vi "encoder_test_3mode_2motor_2.vi"() -> ()   [LabVIEW 2014]
uses:
  <vilib>/rvi/FXPMathLib/FxpSinAndCos/subVIs/nifxpmath_SinAndCos_SimConfig.ctl
  <vilib>/rvi/Emulation/niFpgaGetClockAttributes.vi
  <vilib>/rvi/Emulation/niFpgaSctlEmulationGetInTimedLoop.vi
  <vilib>/rvi/Emulation/niFpgaEmulationReportErrorSimple.vi
  <vilib>/rvi/eio/common/nirviEmuTemplateMethod_errors.vi
  <vilib>/rvi/Emulation/niFpgaProcessEmulError.vi
  <vilib>/rvi/Emulation/niFpgaCriticalErrorInLSC.vi
  <vilib>/rvi/FXPMathLib/FxpSinAndCos/simVIs/DllFxpSinAndCosTemp_sub.vi
  <vilib>/rvi/interface/RandomDataEmulation/nirviRandomDataMultiElementFPGAFIFO.vi
  <instcachedir>/0/nirviRandomDataMultiElementFPGAFIFO_AD0CFC12EF974623A9C2E4184BC062B2.lvgen/nirviRandomDataMultiElementFPGAFIFO_AD0CFC12EF974623A9C2E4184BC062B2_023.vi
  <vilib>/rvi/interface/RandomDataEmulation/niFpgaRandomDataHandleErrors.vi
  <vilib>/eio/EIONode/EIONode.xnode
  <vilib>/rvi/FXPMathLib/FxpMul/XNode/nifxpmath_Multiplier.xnode
  <vilib>/rvi/FXPMathLib/FxpSinAndCos/XNode/nifxpmath_SinAndCos.xnode
  <vilib>/rvi/Analysis/measure/butterworth/XNode/niFpgaButterworthFilter.xnode
  <vilib>/rvi/FXPMathLib/FxpSub/XNode/nifxpmath_Sub.xnode
  <vilib>/rvi/FXPMathLib/FxpAdd/XNode/nifxpmath_Add.xnode
  <vilib>/rvi/DataTransferAndStorage/Container/XNode/niFpgaContainer.xnode
  <vilib>/rvi/interface/RandomDataEmulation/nirviRandomDataFpgaMultiElementTemplate.vi
  <vilib>/rvi/FXPMathLib/sim/FxpSim.dll
panel:
  in  "mt0_y":u32
  out "Dyr_sin_dd":fxp<+/-,64,25>
  out "Dyr_sin_d":fxp<+/-,64,16>
  out "Dyr_sin":fxp<+/-,30,11>
  in  "Sin offset_y":fxp<+/-,29,10>
  out "Sin omega_y":fxp<+/-,41,8>
  in  "Sin magnitude_y":fxp<+/-,11,8>
  in  "Sin frequency_y (Hz)":fxp<+/-,21,5>
  out "Dyr_ramp":fxp<+/-,32,7>
  out "Time now_y (s)":fxp<+,52,14>
  out "Dyr_slope":fxp<+/-,32,10>
  in  "Dyr_time":fxp<+/-,32,10>
  in  "Dyr_end":fxp<+/-,32,7>
  out "Dy_i":fxp<+/-,32,10>
  out "Dyr":fxp<+/-,36,11>
  in  "Direction_y":bool
  in  "Command type_y":i16(ring) items=["Step", "Ramp", "Sine"]
  out "Dy_error":fxp<+/-,37,10>
  out "Fmr_y":fxp<+/-,32,10>
  in  "Ki_y":fxp<+/-,20,6>
  in  "Dy_tolorence":fxp<+/-,18,1>
  in  "Kd_y":fxp<+/-,20,8>
  in  "Kp_y":fxp<+/-,20,8>
  in  "scaled coefficients_Dy_dd":i32[](array[numeric])=[780119100, 146811362]
  out "Dy_dd":fxp<+/-,36,10>
  out "va_y":fxp<+/-,38,8>
  out "vb_y":fxp<+/-,38,8>
  out "vd_y":fxp<+/-,20,5>
  out "vq_y":fxp<+/-,20,5> format="%.57g"
  in  "Stop motor_y":bool
  out "Dy_d (mm/s)":fxp<+/-,33,9>
  out "omega_y (rad/s)":fxp<+/-,33,9>
  in  "Velocity Estimation_y":i16(ring) items=["M_avg method", "M method", "T method"]
  out "Dy_d (T)":fxp<+/-,32,8>
  out "mt_y":u32
  out "omega_y (T)":fxp<+/-,20,9>
  out "omega_y (M)":fxp<+/-,32,8>
  out "Dy_d (M)":fxp<+/-,32,8>
  in  "Dy_d_M_Tc (mSec)":u32 format="%#_6f"
  out "omega_y(M_avg)":fxp<+/-,32,8>
  out "Dy_d (M_avg)":fxp<+,32,8>
  in  "Dy_d_M_avg_Tc (uSec)":u32
  out "rad_y(NrTheta)":fxp<+/-,33,18>
  out "Dy (mm)":fxp<+/-,22,8>
  out "Encoder Position_y":i32
  in  "Encoder Reset_y":bool
  out "omega_p (M_avg)":fxp<+/-,32,8>
  out "Dp_d (M_avg)":fxp<+/-,32,8>
  in  "Dp_d_M_avg_Tc (uSec)":u32 caption="D_d_M_avg_Tc (uSec)"
  out "omega_p (M)":fxp<+/-,32,8>
  out "Dp_d (M)":fxp<+/-,32,8>
  in  "Dp_d_M_Tc (mSec)":u32 format="%#_6f"
  out "Dp_d (T)":fxp<+/-,32,8>
  out "omega_p(T)":fxp<+/-,20,9>
  in  "Velocity Estimation_p":i16(ring) items=["M_avg method", "M method", "T method"]
  out "Dpr_ramp":fxp<+/-,32,7>
  out "Dpr_slope":fxp<+/-,32,10>
  in  "Dpr_time":fxp<+/-,32,10>
  out "Dpr_sin":fxp<+/-,30,11>
  out "Dpr_sin_d":fxp<+/-,64,16>
  out "Dpr_sin_dd":fxp<+/-,64,25>
  out "Sin omega_p":fxp<+/-,41,8>
  in  "Sin offset_p":fxp<+/-,27,10>
  in  "Sin magnitude_p":fxp<+/-,11,8>
  in  "Sin frequency_p (Hz)":fxp<+/-,21,5>
  out "Time now_p (s)":fxp<+,52,14>
  out "Dpr":fxp<+/-,36,11>
  in  "Dpr_end":fxp<+/-,32,7>
  in  "Command type_p":i16(ring) items=["Step", "Ramp", "Sine"]
  out "Dp_i":fxp<+/-,32,10>
  in  "Dp_tolorence":fxp<+/-,18,1>
  in  "Ki_p":fxp<+/-,20,6>
  out "Dp_error":fxp<+/-,37,10>
  in  "Direction_p":bool
  out "Fmr_p":fxp<+/-,32,10>
  in  "Kd_p":fxp<+/-,20,8>
  in  "Kp_p":fxp<+/-,20,12>
  in  "scaled coefficients_Dp_dd":i32[](array[numeric])=[780119100, 146811362]
  out "Dp_dd":fxp<+/-,36,10>
  in  "Ini coe.":bool
  out "va_p":fxp<+/-,38,8>
  out "vb_p":fxp<+/-,38,8>
  in  "Stop motor_p":bool
  out "vq_p":fxp<+/-,20,5> format="%.57g"
  out "vd_p":fxp<+/-,20,5>
  out "Dp_d (mm/s)":fxp<+/-,32,8>
  out "mt_p":u32
  out "omega_p (rad/s)":fxp<+/-,33,9>
  in  "mt0_p":u32
  out "Dp (mm)":fxp<+/-,22,8>
  out "rad_p(NrTheta)":fxp<+/-,33,18>
  out "Encoder Position_p":i32
  in  "Encoder Reset_p":bool
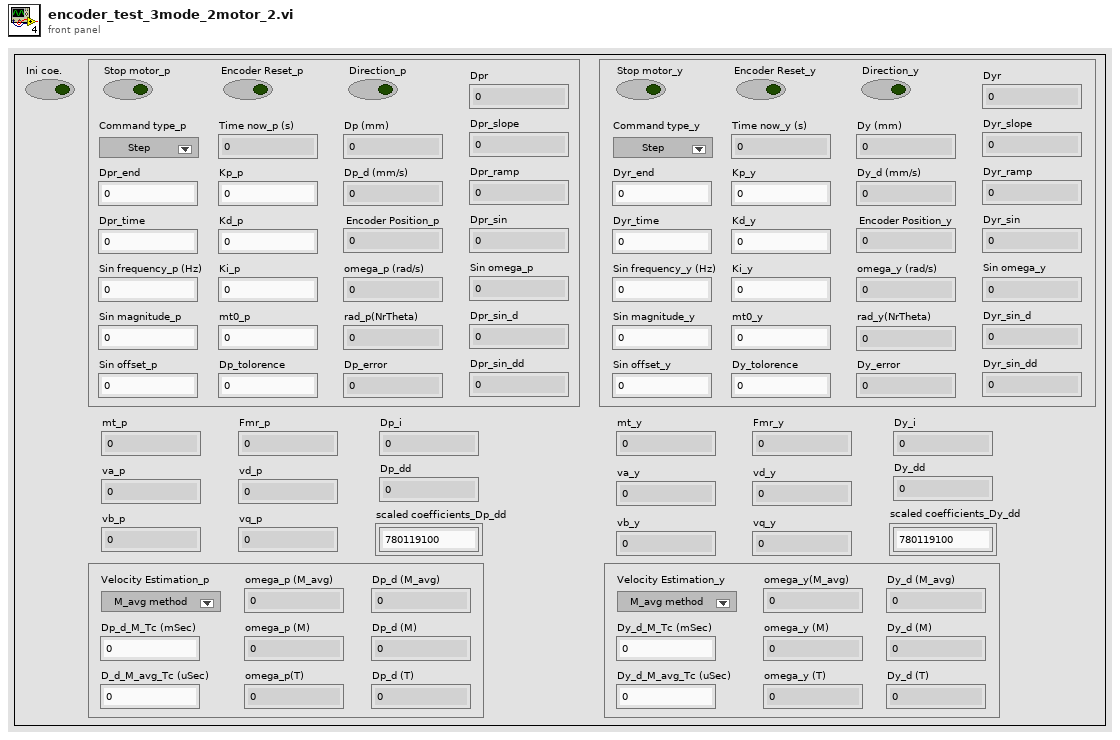
[diagram p1: front panel]
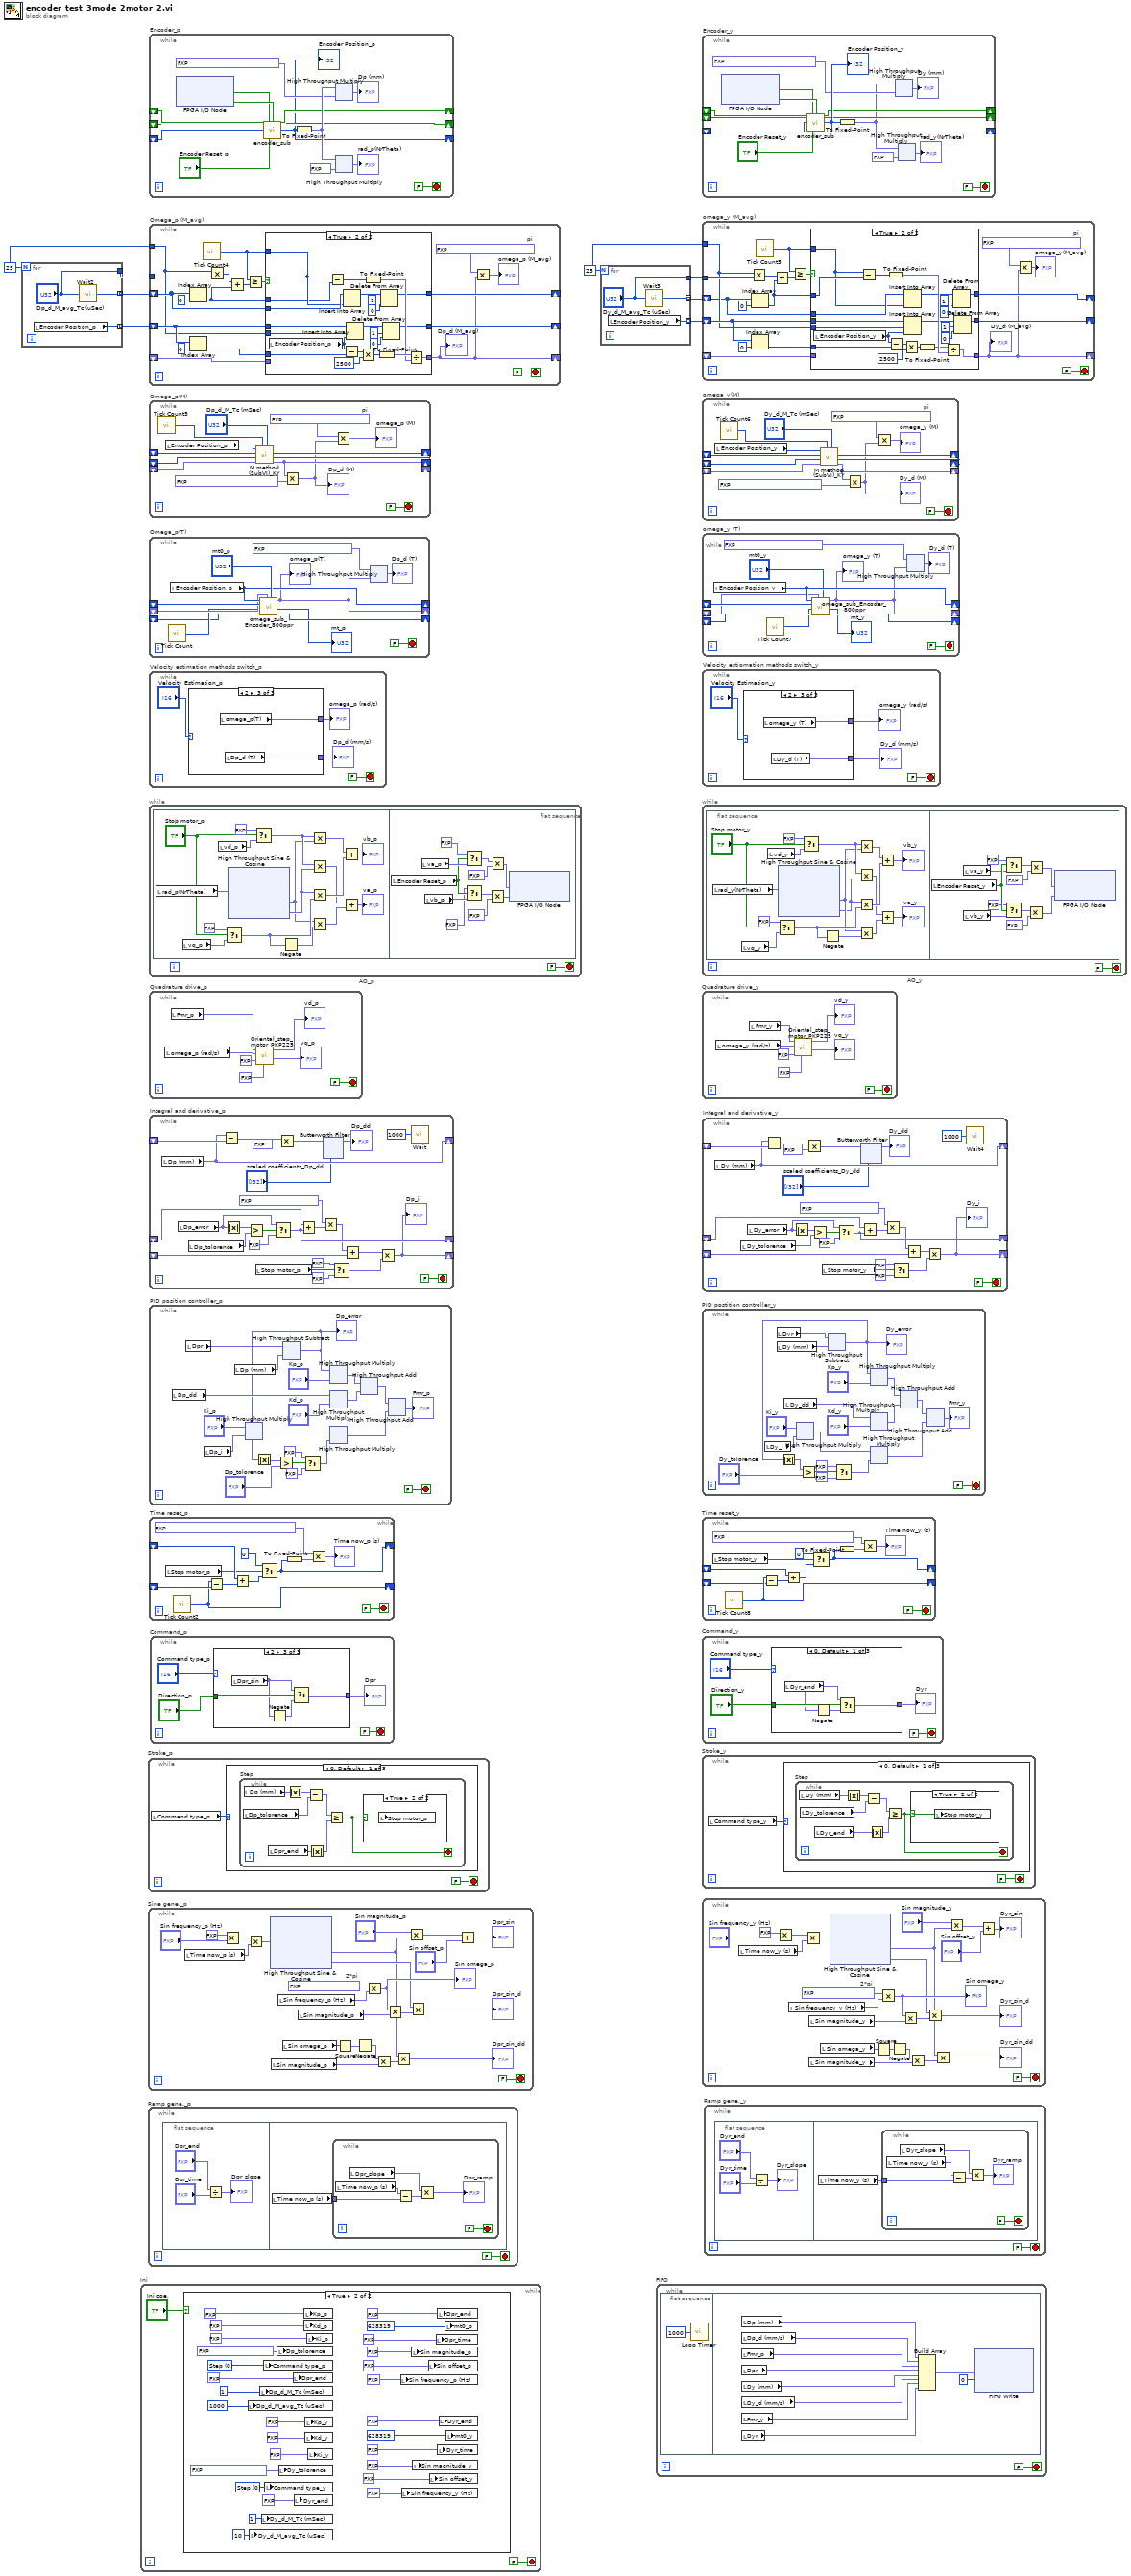
[diagram p0: block diagram]
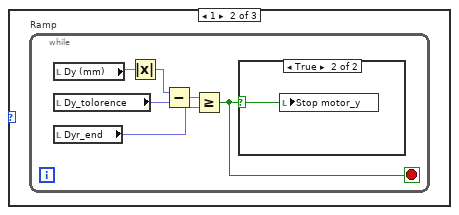
[diagram p3: hidden frame]
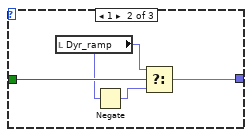
[diagram p6: hidden frame]
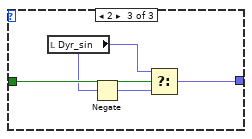
[diagram p7: hidden frame]
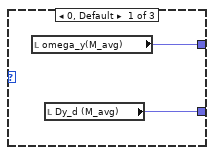
[diagram p8: hidden frame]
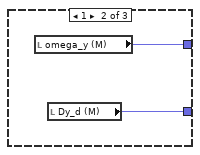
[diagram p9: hidden frame]
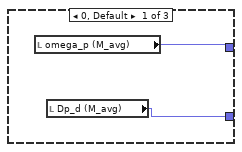
[diagram p12: hidden frame]
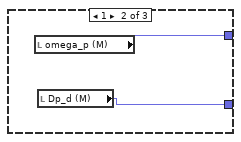
[diagram p13: hidden frame]
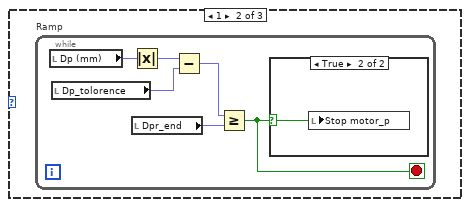
[diagram p15: hidden frame]
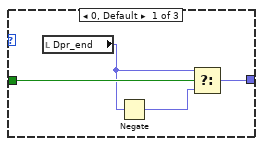
[diagram p18: hidden frame]
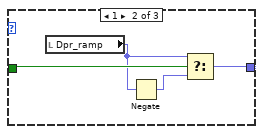
[diagram p19: hidden frame]
diagram:
  w4 = 25
  w8 = 25
  n1 = for {
    N: w8 -> [_]
    tunnel: ["Dp_d_M_avg_Tc (uSec)"] -> w5
    tunnel: [w10] -> w7 mode=indexing
    tunnel: [w9] -> w6 mode=indexing
    n2 = local read "Encoder Position_p"() -> (w9:i32)
    n3 = call "Wait2"("Count(uSec)"="Dp_d_M_avg_Tc (uSec)") -> ("Tick Count(uSec)"=w10:u32)
  }
  n4 = while "Ini" {
    stop <- FALSE stop-if-true
    n5 = case shown="True" "Ini coe." {
      frame False {
      }
      frame True {
        w23 = i16 0 items=["Step", "Ramp", "Sine"] ("Command type_y")
        w35 = i16 0 items=["Step", "Ramp", "Sine"] ("Command type")
        n6 = local write "Dp_d_M_avg_Tc (uSec)"(u32 1000 ("D_d_M_avg_Tc (uSec)")) -> ()
        n7 = local write "Dy_d_M_avg_Tc (uSec)"(u32 10 ("Dy_d_M_avg_Tc (uSec)")) -> ()
        n8 = local write "Dp_d_M_Tc (mSec)"(u32 1 ("D_d_M_Tc (uSec)")) -> ()
        n9 = local write "Dy_d_M_Tc (mSec)"(u32 1 ("Dy_d_M_Tc (mSec)")) -> ()
        n10 = local write "Command type_p"(w35) -> ()
        n11 = local write "Command type_y"(w23) -> ()
        n12 = local write "Dp_tolorence"(fxp<+,18,1> 0.01000213623046875 ("D_tolorence")) -> ()
        n13 = local write "Dy_tolorence"(fxp<+/-,18,1> 0.01000213623046875 ("Dy_tolorence")) -> ()
        n14 = local write "Dpr_end"(fxp<+/-,16,11> 20.0 ("Dr_end")) -> ()
        n15 = local write "Dyr_end"(fxp<+/-,32,7> 20.0 ("Dyr_end")) -> ()
        n16 = local write "Kp_p"(fxp<+/-,20,12> 10.0 ("Kp")) -> ()
        n17 = local write "Kd_p"(fxp<+/-,20,8> 0.0 ("Kd")) -> ()
        n18 = local write "Kp_y"(fxp<+/-,20,8> 10.0 ("Kp_y")) -> ()
        n19 = local write "Kd_y"(fxp<+/-,20,8> 0.0 ("Kd_y")) -> ()
        n20 = local write "Ki_p"(fxp<+/-,20,6> 8.0 ("D_i")) -> ()
        n21 = local write "Ki_y"(fxp<+/-,20,6> 8.0 ("Ki_y")) -> ()
        n22 = local write "Sin frequency_p (Hz)"(fxp<+/-,21,5> 0.5 ("Sin wave frequency (Hz)")) -> ()
        n23 = local write "Sin frequency_y (Hz)"(fxp<+/-,21,5> 0.5 ("Sin frequency_y (Hz)")) -> ()
        n24 = local write "Sin magnitude_p"(fxp<+/-,11,8> 20.0 ("Sin magnitude")) -> ()
        n25 = local write "Sin magnitude_y"(fxp<+/-,11,8> 20.0 ("Sin magnitude_y")) -> ()
        n26 = local write "Sin offset_p"(fxp<+/-,27,10> 0.0 ("Sin offset")) -> ()
        n27 = local write "Sin offset_y"(fxp<+/-,29,10> 0.0 ("Sin offset_y")) -> ()
        n28 = local write "Dpr_time"(fxp<+/-,16,11> 5.0 ("Dr_time")) -> ()
        n29 = local write "Dyr_time"(fxp<+/-,32,10> 10.0 ("Dyr_time")) -> ()
        n30 = local write "Dpr_end"(fxp<+/-,11,7> 20.0 ("Fmr")) -> ()
        n31 = local write "Dyr_end"(fxp<+/-,32,7> 20.0 ("Dyr_end")) -> ()
        n32 = local write "mt0_p"(u32 628319 ("mt0")) -> ()
        n33 = local write "mt0_y"(u32 628319 ("mt0_y")) -> ()
      }
    }
  }
  n34 = while "Stroke_p" {
    stop <- FALSE stop-if-true
    n35 = local read "Command type_p"() -> (w43:i16)
    n36 = case shown="0, Default" w43 {
      frame 0, Default {
        n37 = while "Step" {
          stop <- w44 stop-if-true
          n38 = local read "Dp_tolorence"() -> (w46:fxp<+/-,18,1>)
          n39 = local read "Dp (mm)"() -> (w48:fxp<+/-,22,8>)
          n40 = local read "Dpr_end"() -> (w50:fxp<+/-,32,7>)
          n41 = Absolute Value(x=w48) -> (abs(x)=w47:fxp<+,22,8>)
          n42 = Subtract(x=w47, y=w46) -> (x-y=w45:fxp<+/-,26,9>)
          n43 = Absolute Value(x=w50) -> (abs(x)=w49:fxp<+,32,7>)
          n44 = Greater Or Equal?(x=w45, y=w49) -> (x >= y?=w44:bool)
          n45 = case shown="True" w44 {
            selector: w44 -> [_ w51]
            frame False {
            }
            frame True {
              n46 = local write "Stop motor_p"(w51) -> ()
            }
          }
        }
      }
      frame 1 {
        n47 = while "Ramp" {
          stop <- w52 stop-if-true
          n48 = local read "Dp (mm)"() -> (w54:fxp<+/-,22,8>)
          n49 = local read "Dp_tolorence"() -> (w56:fxp<+/-,18,1>)
          n50 = Absolute Value(x=w54) -> (abs(x)=w55:fxp<+,22,8>)
          n51 = local read "Dpr_end"() -> (w53:fxp<+/-,32,7>)
          n52 = Subtract(x=w55, y=w56) -> (x-y=w57:fxp<+/-,26,9>)
          n53 = Greater Or Equal?(x=w57, y=w53) -> (x >= y?=w52:bool)
          n54 = case shown="True" w52 {
            selector: w52 -> [_ w58]
            frame False {
            }
            frame True {
              n55 = local write "Stop motor_p"(w58) -> ()
            }
          }
        }
      }
      frame 2 {
      }
    }
  }
  n56 = while "Sine gene._p" {
    stop <- FALSE stop-if-true
    w76 = fxp<+,20,3> 6.2831878662109375  # 2*pi
    n57 = local read "Time now_p (s)"() -> (w79:fxp<+,52,14>)
    n58 = Multiply(x=fxp<+,1,2> 2.0, y="Sin frequency_p (Hz)") -> (x*y=w80:fxp<+/-,21,6>)
    n59 = Multiply(x=w80, y=w79) -> (x*y=w60:fxp<+/-,64,20>)
    n60 = xnode "High Throughput Sine & Cosine"("x (pi)"=w60) -> ("sin(x)"=w64:fxp<+/-,18,2>, "cos(x)"=w71:fxp<+/-,18,2>)
    n61 = local read "Sin magnitude_p"() -> (w66:fxp<+/-,11,8>)
    n62 = local read "Sin frequency_p (Hz)"() -> (w75:fxp<+/-,21,5>)
    n63 = local read "Sin omega_p"() -> (w67:fxp<+/-,41,8>)
    n64 = local read "Sin magnitude_p"() -> (w70:fxp<+/-,11,8>)
    n65 = Square(x=w67) -> (x^2=w68:fxp<+,64,14>)
    n66 = Negate(x=w68) -> (-x=w65:fxp<+/-,64,15>)
    n67 = Multiply(x=w76, y=w75) -> (x*y=w72:fxp<+/-,41,8>)
    "Sin omega_p" <- w72
    n68 = Multiply(x=w65, y=w66) -> (x*y=w69:fxp<+/-,64,23>)
    n69 = Multiply(x=w72, y=w70) -> (x*y=w77:fxp<+/-,51,15>)
    n70 = Multiply(x=w64, y=w69) -> (x*y=→"Dpr_sin_dd":fxp<+/-,64,25>)
    n71 = Multiply(x="Sin magnitude_p", y=w64) -> (x*y=w78:fxp<+/-,29,10>)
    n72 = Multiply(x=w71, y=w77) -> (x*y=→"Dpr_sin_d":fxp<+/-,64,16>)
    n73 = Add(x=w78, y="Sin offset_p") -> (x+y=→"Dpr_sin":fxp<+/-,30,11>)
  }
  n74 = while "Ramp gene._p" {
    stop <- FALSE stop-if-true
    n75 = flat-sequence {
      frame #0 {
        n76 = Divide(x="Dpr_end", y="Dpr_time") -> (x/y=→"Dpr_slope":fxp<+/-,64,30>)
      }
      frame #1 {
        n77 = local read "Time now_p (s)"() -> (w117:fxp<+,52,14>)
        n78 = while {
          tunnel: w117 -> [w123]
          stop <- FALSE stop-if-true
          n79 = local read "Time now_p (s)"() -> (w120:fxp<+,52,14>)
          n80 = local read "Dpr_slope"() -> (w121:fxp<+/-,32,10>)
          n81 = Subtract(x=w120, y=w123) -> (x-y=w122:fxp<+/-,53,15>)
          n82 = Multiply(x=w121, y=w122) -> (x*y=→"Dpr_ramp":fxp<+/-,64,24>)
        }
      }
    }
  }
  n83 = while "Encoder_p" {
    shift-right: [w130] -> _
    shift-left: _ -> [w132]
    shift-right: [w129] -> _
    shift-left: _ -> [w131]
    shift-right: [w127] -> _
    shift-left: _ -> [w128]
    stop <- FALSE stop-if-true
    n84 = xnode "FPGA I/O Node"() -> ("Mod4/DI3"=w137:bool, "Mod4/DI4"=w138:bool)  [unwired: 2 in, 2 out]
    n85 = call "encoder_sub.vi"("A_pre"=w132, "B_pre"=w131, "Encoder Position_pre"=w128, "A input"=w137, "Encoder Position Reset"="Encoder Reset_p", "B input"=w138) -> ("A"=w130:bool, "B"=w129:bool, "Encoder Position (Counts)"=w127:i32)  [unwired: 19 in]
    "Encoder Position_p" <- w127
    n86 = To Fixed-Point(number=w127) -> (fixed-point=w135:fxp<+/-,32,32>)  [unwired: 1 in]
    n87 = xnode ("High Throughput Multiply")("x"=w135, "y"=fxp<+/-,24,0> 0.002499997615814209) -> ("x*y"=→"Dp (mm)":fxp<+/-,56,32>)
    n88 = xnode ("High Throughput Multiply")("x"=w135, "y"=fxp<+/-,24,0> 0.125) -> ("x*y"=→"rad_p(NrTheta)":fxp<+/-,56,32>)
  }
  n89 = while "Omega_p (M_avg)" {
    tunnel: w8 -> [w150]
    shift-right: [w143] -> _
    shift-left: w7 -> [w154]
    shift-right: [w142] -> _
    shift-left: _ -> [w145]
    shift-right: [w144] -> _
    shift-left: w6 -> [w153]
    tunnel: w5 -> [w147]
    stop <- FALSE stop-if-true
    w141 = fxp<+/-,27,3> 3.1415926218032837  # pi
    n90 = Index Array(array=w154, index=0) -> (element=w148:u32)
    n91 = Index Array(array=w153, index=0) -> (element=w149:i32)
    n92 = call "Tick Count4"() -> ("Tick Count(uSec)"=w151:u32)
    n93 = Multiply(x=w150, y=w147) -> (x*y=w155:u32)
    n94 = Add(x=w155, y=w148) -> (x+y=w152:u32)
    n95 = Greater Or Equal?(x=w151, y=w152) -> (x >= y?=w146:bool)
    n96 = case shown="True" w146 {
      tunnel: w154 -> [w160 w177]
      tunnel: w153 -> [w159 w176]
      tunnel: w151 -> [_ w169]
      tunnel: w150 -> [_ w175]
      tunnel: w149 -> [_ w173]
      tunnel: w148 -> [_ w168]
      tunnel: w145 -> [w158 _]
      tunnel: [w159 w163] -> w144
      tunnel: [w160 w162] -> w143
      tunnel: [w158 w161] -> w142
      frame False {
      }
      frame True {
        n97 = local read "Encoder Position_p"() -> (w174:i32)
        n98 = Subtract(x=w169, y=w168) -> (x-y=w166:u32)
        n99 = Insert Into Array(array=w177, new element=w169) -> (w178:u32[])  [unwired: 1 in]
        n100 = Subtract(x=w174, y=w173) -> (x-y=w172:i32)
        n101 = Insert Into Array(array=w176, index=w175, new element=w174) -> (w179:i32[])
        n102 = Multiply(x=w172, y=2500) -> (x*y=w170:i32)
        n103 = To Fixed-Point(number=w166) -> (fixed-point=w164:fxp<+,32,32>)  [unwired: 1 in]
        n104 = To Fixed-Point(number=w170) -> (fixed-point=w165:fxp<+/-,32,32>)  [unwired: 1 in]
        n105 = Delete From Array(array=w178, length=1, index=0) -> (array with subset deleted=w162:u32[])  [unwired: 1 out]
        n106 = Delete From Array(array=w179, length=1, index=0) -> (array with subset deleted=w163:i32[])  [unwired: 1 out]
        n107 = Divide(x=w165, y=w164) -> (x/y=w161:fxp<+/-,64,32>)
      }
    }
    "Dp_d (M_avg)" <- w142
    n108 = Multiply(x=w141, y=w142) -> (x*y=→"omega_p (M_avg)":fxp<+/-,64,35>)
  }
  n109 = while "Omega_p(M)" {
    shift-right: [w194] -> _
    shift-left: _ -> [w195]
    shift-right: [w190] -> _
    shift-left: _ -> [w191]
    shift-right: [w188] -> _
    shift-left: _ -> [w189]
    stop <- FALSE stop-if-true
    w185 = fxp<+/-,27,3> 3.1415926218032837  # pi
    n110 = call "Tick Count3"() -> ("Tick Count(mSec)"=w193:u32)
    n111 = local read "Encoder Position_p"() -> (w196:i32)
    n112 = call "M method (SubVI)_KY.vi"("Tc (mSec)"="Dp_d_M_Tc (mSec)", "Tick Count (mSec)"=w193, "Encoder velocity_pre (pulse/s)"=w189, "Shift Register in 2"=w191, "Shift Register in 1"=w195, "Encoder pulses"=w196) -> ("Encoder velocity (pulse/s)"=w188:fxp<+/-,64,32>, "Shift Register out 2"=w190:i32, "Shift Register out 1"=w194:u32)  [unwired: 3 in]
    n113 = Multiply(x=w188, y=fxp<+/-,20,-5> 0.002499997615814209) -> (x*y=w186:fxp<+/-,64,27>)
    "Dp_d (M)" <- w186
    n114 = Multiply(x=w185, y=w186) -> (x*y=→"omega_p (M)":fxp<+/-,64,30>)
  }
  n115 = while "Omega_p(T)" {
    shift-right: [w206] -> _
    shift-left: _ -> [w207]
    shift-right: [w199] -> _
    shift-left: _ -> [w205]
    shift-right: [w202] -> _
    shift-left: _ -> [w203]
    stop <- FALSE stop-if-true
    n116 = call "Tick Count"() -> ("Tick Count(Ticks)"=w204:u32)
    n117 = local read "Encoder Position_p"() -> (w206:i32)
    n118 = call "omega_sub_Encoder_800ppr.vi"("mt0"="mt0_p", "omega_pre"=w205, "ticks_m_pre"=w203, "ticks"=w204, "count_pre"=w207, "count"=w206) -> ("ticks_m"=w202:u32, "mt"=→"mt_p":u32, "omega"=w199:fxp<+/-,20,9>)  [unwired: 3 in]
    "omega_p(T)" <- w199
    n119 = xnode ("High Throughput Multiply")("x"=fxp<+/-,26,1> 0.3183099031448364, "y"=w199) -> ("x*y"=→"Dp_d (T)":fxp<+/-,46,10>)
  }
  n120 = while "Velocity estimation methods switch_p" {
    stop <- FALSE stop-if-true
    n121 = case shown="2" "Velocity Estimation_p" {
      tunnel: [w214 w216 w218] -> w211
      tunnel: [w213 w215 w217] -> w210
      frame 0, Default {
        n122 = local read "omega_p (M_avg)"() -> (w214:fxp<+/-,32,8>)
        n123 = local read "Dp_d (M_avg)"() -> (w213:fxp<+/-,32,8>)
      }
      frame 1 {
        n124 = local read "omega_p (M)"() -> (w216:fxp<+/-,32,8>)
        n125 = local read "Dp_d (M)"() -> (w215:fxp<+/-,32,8>)
      }
      frame 2 {
        n126 = local read "omega_p(T)"() -> (w218:fxp<+/-,20,9>)
        n127 = local read "Dp_d (T)"() -> (w217:fxp<+/-,32,8>)
      }
    }
    "Dp_d (mm/s)" <- w210
    "omega_p (rad/s)" <- w211
  }
  n128 = while "AO_p" {
    stop <- FALSE stop-if-true
    n129 = flat-sequence {
      frame #0 {
        n130 = local read "rad_p(NrTheta)"() -> (w235:fxp<+/-,33,18>)
        n131 = local read "vq_p"() -> (w233:fxp<+/-,20,5>)
        n132 = local read "vd_p"() -> (w234:fxp<+/-,20,5>)
        n133 = Select(t=fxp<+,20,5> 0.0, s="Stop motor_p", f=w233) -> (s? t:f=w230:fxp<+/-,21,6>)
        n134 = xnode "High Throughput Sine & Cosine"("x (pi)"=w235) -> ("sin(x)"=w226:fxp<+/-,17,2>, "cos(x)"=w228:fxp<+/-,17,2>)
        n135 = Select(t=fxp<+,20,5> 0.0, s="Stop motor_p", f=w234) -> (s? t:f=w227:fxp<+/-,21,6>)
        n136 = Negate(x=w230) -> (-x=w229:fxp<+/-,21,6>)
        n137 = Multiply(x=w227, y=w226) -> (x*y=w225:fxp<+/-,37,7>)
        n138 = Multiply(x=w227, y=w228) -> (x*y=w223:fxp<+/-,37,7>)
        n139 = Multiply(x=w228, y=w230) -> (x*y=w224:fxp<+/-,37,7>)
        n140 = Multiply(x=w226, y=w229) -> (x*y=w222:fxp<+/-,37,7>)
        n141 = Add(x=w225, y=w224) -> (x+y=→"vb_p":fxp<+/-,38,8>)
        n142 = Add(x=w223, y=w222) -> (x+y=→"va_p":fxp<+/-,38,8>)
      }
      frame #1 {
        n143 = local read "Encoder Reset_p"() -> (w269:bool)
        n144 = local read "va_p"() -> (w271:fxp<+/-,38,8>)
        n145 = local read "vb_p"() -> (w270:fxp<+/-,38,8>)
        n146 = Select(t=fxp<+/-,20,5> 5.0 ("y"), s=w269, f=w271) -> (s? t:f=w272:fxp<+/-,38,8>)
        n147 = Select(t=fxp<+/-,20,5> 0.0 ("y"), s=w269, f=w270) -> (s? t:f=w273:fxp<+/-,38,8>)
        n148 = Multiply(x=w273, y=fxp<+/-,20,5> -0.5) -> (x*y=w277:fxp<+/-,57,12>)
        n149 = Multiply(x=w272, y=fxp<+/-,20,5> -0.5) -> (x*y=w276:fxp<+/-,57,12>)
        n150 = xnode "FPGA I/O Node"("Mod8/AO0"=w276, "Mod8/AO1"=w277) -> ()  [unwired: 2 in, 2 out]
      }
    }
  }
  n151 = while "Quadrature drive_p" {
    stop <- FALSE stop-if-true
    n152 = local read "omega_p (rad/s)"() -> (w280:fxp<+/-,33,9>)
    n153 = local read "Fmr_p"() -> (w278:fxp<+/-,32,10>)
    n154 = call "Oriental_step_motor_PKP225.vi"("F_Threshold"=fxp<+,12,12> 10.0, "dFmr"=fxp<+/-,25,15> 0.0, "omega"=w280, "Fmr"=w278) -> ("vq_F"=→"vq_p":fxp<+/-,20,5>, "vd_F"=→"vd_p":fxp<+/-,20,5>)  [unwired: 6 in]
  }
  n155 = while "Integral and derivative_p" {
    shift-right: [w305] -> _
    shift-left: _ -> [w309]
    shift-right: [w295] -> _
    shift-left: _ -> [w296]
    shift-right: [w285] -> _
    shift-left: _ -> [w289]
    stop <- FALSE stop-if-true
    n156 = local read "Dp (mm)"() -> (w305:fxp<+/-,22,8>)
    n157 = local read "Dp_error"() -> (w297:fxp<+/-,37,10>)
    n158 = local read "Dp_tolorence"() -> (w300:fxp<+/-,18,1>)
    n159 = Subtract(x=w305, y=w309) -> (x-y=w308:fxp<+/-,23,9>)
    n160 = Absolute Value(x=w297) -> (abs(x)=w301:fxp<+,37,10>)
    n161 = Greater?(x=w301, y=w300) -> (0:w299:bool)
    n162 = local read "Stop motor_p"() -> (w292:bool)
    n163 = Select(t=w297, s=w299, f=fxp<+,24,11> 0.0) -> (s? t:f=w295:fxp<+/-,39,12>)
    n164 = Multiply(x=w308, y=fxp<+/-,33,13> 1000.0) -> (x*y=w306:fxp<+/-,55,21>)
    n165 = Add(x=w296, y=w295) -> (x+y=w294:fxp<+/-,40,13>)
    n166 = Multiply(x=fxp<+/-,30,12> 0.000499725341796875, y=w294) -> (x*y=w288:fxp<+/-,64,24>)
    n167 = xnode "Butterworth Filter"("input data"=w306, "scaled coefficients"="scaled coefficients_Dp_dd") -> ("output data"=→"Dp_dd":fxp<+/-,36,25>)  [unwired: 1 in]
    n168 = Select(t=fxp<+,1,1> 0.0, s=w292, f=fxp<+,1,1> 1.0) -> (s? t:f=w286:fxp<+,1,1>)
    n169 = Add(x=w288, y=w289) -> (x+y=w287:fxp<+/-,32,16>)
    n170 = Multiply(x=w287, y=w286) -> (x*y=w285:fxp<+/-,32,16>)
    "Dp_i" <- w285
    n171 = call "Wait"("Count(uSec)"=u32 1000) -> ()  [unwired: 1 out]
  }
  n172 = while "PID position controller_p" {
    stop <- FALSE stop-if-true
    n173 = local read "Dp_dd"() -> (w335:fxp<+/-,36,10>)
    n174 = local read "Dpr"() -> (w319:fxp<+/-,36,11>)
    n175 = local read "Dp_i"() -> (w330:fxp<+/-,32,10>)
    n176 = local read "Dp (mm)"() -> (w339:fxp<+/-,22,8>)
    n177 = xnode ("High Throughput Multiply")("x"="Ki_p", "y"=w330) -> ("x*y"=w324:fxp<+/-,52,16>)
    n178 = xnode "High Throughput Subtract"("x"=w319, "y"=w339) -> ("x-y"=w328:fxp<+/-,37,12>)
    "Dp_error" <- w328
    n179 = Absolute Value(x=w328) -> (abs(x)=w329:fxp<+,37,12>)
    n180 = Greater?(x=w329, y="Dp_tolorence") -> (0:w327:bool)
    n181 = Select(t=fxp<+,10,2> 1.0, s=w327, f=fxp<+,10,2> 0.0) -> (s? t:f=w323:fxp<+,10,2>)
    n182 = xnode ("High Throughput Multiply")("x"=w324, "y"=w323) -> ("x*y"=w320:fxp<+/-,62,18>)
    n183 = xnode ("High Throughput Multiply")("x"=w328, "y"="Kp_p") -> ("x*y"=w337:fxp<+/-,57,24>)
    n184 = xnode ("High Throughput Multiply")("x"=w335, "y"="Kd_p") -> ("x*y"=w336:fxp<+/-,56,18>)
    n185 = xnode ("High Throughput Add")("x"=w337, "y"=w336) -> ("x+y"=w321:fxp<+/-,63,25>)
    n186 = xnode ("High Throughput Add")("x"=w321, "y"=w320) -> ("x+y"=→"Fmr_p":fxp<+/-,64,26>)
  }
  n187 = while "Time reset_p" {
    shift-right: [w343] -> _
    shift-left: _ -> [w350]
    shift-right: [w345] -> _
    shift-left: _ -> [w346]
    stop <- FALSE stop-if-true
    n188 = local read "Stop motor_p"() -> (w348:bool)
    n189 = call "Tick Count2"() -> ("Tick Count(uSec)"=w345:u32)
    n190 = Subtract(x=w345, y=w346) -> (x-y=w351:u32)
    n191 = Add(x=w350, y=w351) -> (x+y=w349:u32)
    n192 = Select(t=u32 0, s=w348, f=w349) -> (s? t:f=w343:u32)
    n193 = To Fixed-Point(number=w343) -> (fixed-point=w342:fxp<+,32,32>)  [unwired: 1 in]
    n194 = Multiply(x=fxp<+,20,-18> 1.0000003385357559e-06, y=w342) -> (x*y=→"Time now_p (s)":fxp<+,52,14>)
  }
  n195 = while "Command_p" {
    stop <- FALSE stop-if-true
    n196 = case shown="2" "Command type_p" {
      tunnel: [w356 w360 w364] -> w354
      tunnel: "Direction_p" -> [w359 w363 w367]
      frame 0, Default {
        n197 = local read "Dpr_end"() -> (w358:fxp<+/-,32,7>)
        n198 = Negate(x=w358) -> (-x=w357:fxp<+/-,33,8>)
        n199 = Select(t=w358, s=w359, f=w357) -> (s? t:f=w356:fxp<+/-,33,8>)
      }
      frame 1 {
        n200 = local read "Dpr_ramp"() -> (w361:fxp<+/-,32,7>)
        n201 = Negate(x=w361) -> (-x=w362:fxp<+/-,33,8>)
        n202 = Select(t=w361, s=w363, f=w362) -> (s? t:f=w360:fxp<+/-,33,8>)
      }
      frame 2 {
        n203 = local read "Dpr_sin"() -> (w365:fxp<+/-,30,11>)
        n204 = Negate(x=w365) -> (-x=w366:fxp<+/-,29,10>)
        n205 = Select(t=w365, s=w367, f=w366) -> (s? t:f=w364:fxp<+/-,30,11>)
      }
    }
    "Dpr" <- w354
  }
  n206 = for {
    N: w4 -> [_]
    tunnel: ["Dy_d_M_avg_Tc (uSec)"] -> w3
    tunnel: [w369] -> w1 mode=indexing
    tunnel: [w368] -> w2 mode=indexing
    n207 = local read "Encoder Position_y"() -> (w368:i32)
    n208 = call "Wait3"("Count(uSec)"="Dy_d_M_avg_Tc (uSec)") -> ("Tick Count(uSec)"=w369:u32)
  }
  n209 = while "FIFO" {
    stop <- FALSE stop-if-true
    n210 = flat-sequence {
      frame #0 {
        n211 = call "Loop Timer"("Count(uSec)"=u32 1000) -> ()  [unwired: 1 out]
      }
      frame #1 {
        n212 = local read "Dp (mm)"() -> (w380:fxp<+/-,22,8>)
        n213 = local read "Dp_d (mm/s)"() -> (w379:fxp<+/-,32,8>)
        n214 = local read "Fmr_p"() -> (w378:fxp<+/-,32,10>)
        n215 = local read "Dpr"() -> (w377:fxp<+/-,36,11>)
        n216 = local read "Dy (mm)"() -> (w373:fxp<+/-,22,8>)
        n217 = local read "Dy_d (mm/s)"() -> (w376:fxp<+/-,33,9>)
        n218 = local read "Fmr_y"() -> (w375:fxp<+/-,32,10>)
        n219 = local read "Dyr"() -> (w374:fxp<+/-,36,11>)
        n220 = Build Array(w380, w379, w378, w377, w373, w376, w375, w374) -> (w381:fxp<+/-,36,11>[])
        n221 = xnode ("FIFO Write")("Element"=w381, "Timeout"=0) -> ()  [unwired: 1 in, 2 out]
      }
    }
  }
  n222 = while "AO_y" {
    stop <- FALSE stop-if-true
    n223 = flat-sequence {
      frame #0 {
        n224 = local read "rad_y(NrTheta)"() -> (w395:fxp<+/-,33,18>)
        n225 = local read "vq_y"() -> (w398:fxp<+/-,20,5>)
        n226 = local read "vd_y"() -> (w397:fxp<+/-,20,5>)
        n227 = xnode "High Throughput Sine & Cosine"("x (pi)"=w395) -> ("sin(x)"=w391:fxp<+/-,17,2>, "cos(x)"=w390:fxp<+/-,17,2>)
        n228 = Select(t=fxp<+,20,5> 0.0, s="Stop motor_y", f=w398) -> (s? t:f=w393:fxp<+/-,21,6>)
        n229 = Select(t=fxp<+/-,20,5> 0.0, s="Stop motor_y", f=w397) -> (s? t:f=w392:fxp<+/-,20,5>)
        n230 = Negate(x=w393) -> (-x=w394:fxp<+/-,21,6>)
        n231 = Multiply(x=w392, y=w391) -> (x*y=w389:fxp<+/-,37,7>)
        n232 = Multiply(x=w392, y=w390) -> (x*y=w387:fxp<+/-,37,7>)
        n233 = Multiply(x=w390, y=w393) -> (x*y=w388:fxp<+/-,37,7>)
        n234 = Multiply(x=w391, y=w394) -> (x*y=w386:fxp<+/-,37,7>)
        n235 = Add(x=w389, y=w388) -> (x+y=→"vb_y":fxp<+/-,38,8>)
        n236 = Add(x=w387, y=w386) -> (x+y=→"va_y":fxp<+/-,38,8>)
      }
      frame #1 {
        n237 = local read "Encoder Reset_y"() -> (w441:bool)
        n238 = local read "va_y"() -> (w440:fxp<+/-,38,8>)
        n239 = local read "vb_y"() -> (w439:fxp<+/-,38,8>)
        n240 = Select(t=fxp<+/-,20,5> 5.0, s=w441, f=w440) -> (s? t:f=w436:fxp<+/-,38,8>)
        n241 = Select(t=fxp<+/-,20,5> 0.0, s=w441, f=w439) -> (s? t:f=w435:fxp<+/-,38,8>)
        n242 = Multiply(x=w435, y=fxp<+/-,20,5> -0.5) -> (x*y=w431:fxp<+/-,57,12>)
        n243 = Multiply(x=w436, y=fxp<+/-,20,5> -0.5) -> (x*y=w432:fxp<+/-,57,12>)
        n244 = xnode "FPGA I/O Node"("Mod8/AO2"=w432, "Mod8/AO3"=w431) -> ()  [unwired: 2 in, 2 out]
      }
    }
  }
  n245 = while "Quadrature drive_y" {
    stop <- FALSE stop-if-true
    n246 = local read "omega_y (rad/s)"() -> (w448:fxp<+/-,33,9>)
    n247 = local read "Fmr_y"() -> (w443:fxp<+/-,32,10>)
    n248 = call "Oriental_step_motor_PKP225.vi"("F_Threshold"=fxp<+,12,12> 10.0, "dFmr"=fxp<+/-,25,15> 0.0, "omega"=w448, "Fmr"=w443) -> ("vq_F"=→"vq_y":fxp<+/-,20,5>, "vd_F"=→"vd_y":fxp<+/-,20,5>)  [unwired: 6 in]
  }
  n249 = while "PID postition controller_y" {
    stop <- FALSE stop-if-true
    n250 = local read "Dy_i"() -> (w450:fxp<+/-,32,10>)
    n251 = local read "Dyr"() -> (w451:fxp<+/-,36,11>)
    n252 = local read "Dy (mm)"() -> (w460:fxp<+/-,22,8>)
    n253 = local read "Dy_dd"() -> (w461:fxp<+/-,36,10>)
    n254 = xnode ("High Throughput Multiply")("x"="Ki_y", "y"=w450) -> ("x*y"=w459:fxp<+/-,52,16>)
    n255 = xnode "High Throughput Subtract"("x"=w451, "y"=w460) -> ("x-y"=w452:fxp<+/-,37,12>)
    "Dy_error" <- w452
    n256 = Absolute Value(x=w452) -> (abs(x)=w453:fxp<+,37,12>)
    n257 = Greater?(x=w453, y="Dy_tolorence") -> (0:w464:bool)
    n258 = Select(t=fxp<+,1,1> 1.0, s=w464, f=fxp<+,1,1> 0.0) -> (s? t:f=w467:fxp<+,1,1>)
    n259 = xnode ("High Throughput Multiply")("x"=w452, "y"="Kp_y") -> ("x*y"=w458:fxp<+/-,57,20>)
    n260 = xnode ("High Throughput Multiply")("x"=w461, "y"="Kd_y") -> ("x*y"=w457:fxp<+/-,56,18>)
    n261 = xnode ("High Throughput Multiply")("x"=w459, "y"=w467) -> ("x*y"=w455:fxp<+/-,52,16>)
    n262 = xnode ("High Throughput Add")("x"=w458, "y"=w457) -> ("x+y"=w456:fxp<+/-,59,21>)
    n263 = xnode ("High Throughput Add")("x"=w456, "y"=w455) -> ("x+y"=→"Fmr_y":fxp<+/-,60,22>)
  }
  n264 = while "Time reset_y" {
    shift-right: [w476] -> _
    shift-left: _ -> [w475]
    shift-right: [w474] -> _
    shift-left: _ -> [w477]
    stop <- FALSE stop-if-true
    n265 = local read "Stop motor_y"() -> (w481:bool)
    n266 = call "Tick Count8"() -> ("Tick Count(uSec)"=w476:u32)
    n267 = Subtract(x=w476, y=w475) -> (x-y=w480:u32)
    n268 = Add(x=w477, y=w480) -> (x+y=w478:u32)
    n269 = Select(t=u32 0, s=w481, f=w478) -> (s? t:f=w474:u32)
    n270 = To Fixed-Point(number=w474) -> (fixed-point=w473:fxp<+,32,32>)  [unwired: 1 in]
    n271 = Multiply(x=fxp<+,20,-18> 1.0000003385357559e-06, y=w473) -> (x*y=→"Time now_y (s)":fxp<+,52,14>)
  }
  n272 = while "Command_y" {
    stop <- FALSE stop-if-true
    n273 = case shown="0, Default" "Command type_y" {
      tunnel: "Direction_y" -> [w489 w493 w496]
      tunnel: [w488 w490 w497] -> w483
      frame 0, Default {
        n274 = local read "Dyr_end"() -> (w486:fxp<+/-,32,7>)
        n275 = Negate(x=w486) -> (-x=w487:fxp<+/-,33,8>)
        n276 = Select(t=w486, s=w489, f=w487) -> (s? t:f=w488:fxp<+/-,33,8>)
      }
      frame 1 {
        n277 = local read "Dyr_ramp"() -> (w491:fxp<+/-,32,7>)
        n278 = Negate(x=w491) -> (-x=w492:fxp<+/-,33,8>)
        n279 = Select(t=w491, s=w493, f=w492) -> (s? t:f=w490:fxp<+/-,33,8>)
      }
      frame 2 {
        n280 = local read "Dyr_sin"() -> (w494:fxp<+/-,30,11>)
        n281 = Negate(x=w494) -> (-x=w495:fxp<+/-,29,10>)
        n282 = Select(t=w494, s=w496, f=w495) -> (s? t:f=w497:fxp<+/-,30,11>)
      }
    }
    "Dyr" <- w483
  }
  n283 = while "Stroke_y" {
    stop <- FALSE stop-if-true
    n284 = local read "Command type_y"() -> (w499:i16)
    n285 = case shown="0, Default" w499 {
      frame 0, Default {
        n286 = while "Step" {
          stop <- w501 stop-if-true
          n287 = local read "Dy (mm)"() -> (w506:fxp<+/-,22,8>)
          n288 = local read "Dy_tolorence"() -> (w504:fxp<+/-,18,1>)
          n289 = local read "Dyr_end"() -> (w500:fxp<+/-,32,7>)
          n290 = Absolute Value(x=w506) -> (abs(x)=w505:fxp<+,22,8>)
          n291 = Subtract(x=w505, y=w504) -> (x-y=w503:fxp<+/-,26,9>)
          n292 = Absolute Value(x=w500) -> (abs(x)=w502:fxp<+,32,7>)
          n293 = Greater Or Equal?(x=w503, y=w502) -> (x >= y?=w501:bool)
          n294 = case shown="True" w501 {
            selector: w501 -> [_ w507]
            frame False {
            }
            frame True {
              n295 = local write "Stop motor_y"(w507) -> ()
            }
          }
        }
      }
      frame 1 {
        n296 = while "Ramp" {
          stop <- w508 stop-if-true
          n297 = local read "Dy (mm)"() -> (w512:fxp<+/-,22,8>)
          n298 = local read "Dy_tolorence"() -> (w511:fxp<+/-,18,1>)
          n299 = local read "Dyr_end"() -> (w509:fxp<+/-,32,7>)
          n300 = Absolute Value(x=w512) -> (abs(x)=w513:fxp<+,22,8>)
          n301 = Subtract(x=w513, y=w511) -> (x-y=w510:fxp<+/-,26,9>)
          n302 = Greater Or Equal?(x=w510, y=w509) -> (x >= y?=w508:bool)
          n303 = case shown="True" w508 {
            selector: w508 -> [_ w514]
            frame False {
            }
            frame True {
              n304 = local write "Stop motor_y"(w514) -> ()
            }
          }
        }
      }
      frame 2 {
      }
    }
  }
  n305 = while {
    stop <- FALSE stop-if-true
    w530 = fxp<+,20,3> 6.2831878662109375  # 2*pi
    n306 = local read "Time now_y (s)"() -> (w537:fxp<+,52,14>)
    n307 = Multiply(x=fxp<+,1,2> 2.0, y="Sin frequency_y (Hz)") -> (x*y=w536:fxp<+/-,21,6>)
    n308 = local read "Sin frequency_y (Hz)"() -> (w529:fxp<+/-,21,5>)
    n309 = Multiply(x=w536, y=w537) -> (x*y=w538:fxp<+/-,64,20>)
    n310 = local read "Sin magnitude_y"() -> (w528:fxp<+/-,11,8>)
    n311 = local read "Sin magnitude_y"() -> (w523:fxp<+/-,11,8>)
    n312 = local read "Sin omega_y"() -> (w524:fxp<+/-,41,8>)
    n313 = xnode "High Throughput Sine & Cosine"("x (pi)"=w538) -> ("sin(x)"=w521:fxp<+/-,18,2>, "cos(x)"=w525:fxp<+/-,18,2>)
    n314 = Square(x=w524) -> (x^2=w532:fxp<+,64,14>)
    n315 = Multiply(x=w530, y=w529) -> (x*y=w527:fxp<+/-,41,8>)
    "Sin omega_y" <- w527
    n316 = Negate(x=w532) -> (-x=w531:fxp<+/-,64,15>)
    n317 = Multiply(x=w527, y=w528) -> (x*y=w526:fxp<+/-,51,15>)
    n318 = Multiply(x=w531, y=w523) -> (x*y=w522:fxp<+/-,64,23>)
    n319 = Multiply(x=w525, y=w526) -> (x*y=→"Dyr_sin_d":fxp<+/-,64,16>)
    n320 = Multiply(x=w521, y=w522) -> (x*y=→"Dyr_sin_dd":fxp<+/-,64,25>)
    n321 = Multiply(x="Sin magnitude_y", y=w521) -> (x*y=w520:fxp<+/-,29,10>)
    n322 = Add(x=w520, y="Sin offset_y") -> (x+y=→"Dyr_sin":fxp<+/-,30,11>)
  }
  n323 = while "Encoder_y" {
    shift-right: [w577] -> _
    shift-left: _ -> [w575]
    shift-right: [w578] -> _
    shift-left: _ -> [w576]
    shift-right: [w581] -> _
    shift-left: _ -> [w580]
    stop <- FALSE stop-if-true
    n324 = xnode "FPGA I/O Node"() -> ("Mod4/DI0"=w582:bool, "Mod4/DI1"=w583:bool)  [unwired: 2 in, 2 out]
    n325 = call "encoder_sub.vi"("A_pre"=w575, "B_pre"=w576, "Encoder Position_pre"=w580, "A input"=w582, "Encoder Position Reset"="Encoder Reset_y", "B input"=w583) -> ("A"=w577:bool, "B"=w578:bool, "Encoder Position (Counts)"=w581:i32)  [unwired: 19 in]
    "Encoder Position_y" <- w581
    n326 = To Fixed-Point(number=w581) -> (fixed-point=w572:fxp<+/-,32,32>)  [unwired: 1 in]
    n327 = xnode ("High Throughput Multiply")("x"=w572, "y"=fxp<+/-,24,0> 0.002499997615814209) -> ("x*y"=→"Dy (mm)":fxp<+/-,56,32>)
    n328 = xnode ("High Throughput Multiply")("x"=w572, "y"=fxp<+/-,16,1> 0.125) -> ("x*y"=→"rad_y(NrTheta)":fxp<+/-,48,33>)
  }
  n329 = while "omega_y (M_avg)" {
    tunnel: w4 -> [w593]
    tunnel: w3 -> [w599]
    shift-right: [w589] -> _
    shift-left: w1 -> [w590]
    shift-right: [w588] -> _
    shift-left: w2 -> [w594]
    shift-right: [w586] -> _
    shift-left: _ -> [w591]
    stop <- FALSE stop-if-true
    w587 = fxp<+/-,27,3> 3.1415926218032837  # pi
    n330 = Multiply(x=w593, y=w599) -> (x*y=w598:u32)
    n331 = Index Array(array=w590, index=0) -> (element=w595:u32)
    n332 = Index Array(array=w594, index=0) -> (element=w592:i32)
    n333 = call "Tick Count5"() -> ("Tick Count(uSec)"=w596:u32)
    n334 = Add(x=w598, y=w595) -> (x+y=w602:u32)
    n335 = Greater Or Equal?(x=w596, y=w602) -> (x >= y?=w597:bool)
    n336 = case shown="True" w597 {
      tunnel: w596 -> [_ w625]
      tunnel: w595 -> [_ w626]
      tunnel: w594 -> [w604 w615]
      tunnel: w593 -> [_ w616]
      tunnel: w592 -> [_ w617]
      tunnel: w591 -> [w603 _]
      tunnel: w590 -> [w605 w627]
      tunnel: [w605 w608] -> w589
      tunnel: [w604 w607] -> w588
      tunnel: [w603 w606] -> w586
      frame False {
      }
      frame True {
        n337 = local read "Encoder Position_y"() -> (w618:i32)
        n338 = Subtract(x=w625, y=w626) -> (x-y=w624:u32)
        n339 = To Fixed-Point(number=w624) -> (fixed-point=w623:fxp<+,32,32>)  [unwired: 1 in]
        n340 = Subtract(x=w618, y=w617) -> (x-y=w619:i32)
        n341 = Multiply(x=w619, y=u32 2500) -> (x*y=w621:u32)
        n342 = Insert Into Array(array=w627, new element=w625) -> (w613:u32[])  [unwired: 1 in]
        n343 = Insert Into Array(array=w615, index=w616, new element=w618) -> (w614:i32[])
        n344 = To Fixed-Point(number=w621) -> (fixed-point=w622:fxp<+,32,32>)  [unwired: 1 in]
        n345 = Divide(x=w622, y=w623) -> (x/y=w606:fxp<+,64,32>)
        n346 = Delete From Array(array=w613, length=1, index=0) -> (array with subset deleted=w608:u32[])  [unwired: 1 out]
        n347 = Delete From Array(array=w614, length=1, index=0) -> (array with subset deleted=w607:i32[])  [unwired: 1 out]
      }
    }
    "Dy_d (M_avg)" <- w586
    n348 = Multiply(x=w587, y=w586) -> (x*y=→"omega_y(M_avg)":fxp<+/-,64,35>)
  }
  n349 = while "omega_y(M)" {
    shift-right: [w634] -> _
    shift-left: _ -> [w638]
    shift-right: [w635] -> _
    shift-left: _ -> [w637]
    shift-right: [w633] -> _
    shift-left: _ -> [w636]
    stop <- FALSE stop-if-true
    w630 = fxp<+/-,27,3> 3.1415926218032837  # pi
    n350 = local read "Encoder Position_y"() -> (w641:i32)
    n351 = call "Tick Count6"() -> ("Tick Count(mSec)"=w640:u32)
    n352 = call "M method (SubVI)_KY.vi"("Tc (mSec)"="Dy_d_M_Tc (mSec)", "Tick Count (mSec)"=w640, "Encoder velocity_pre (pulse/s)"=w636, "Shift Register in 2"=w637, "Shift Register in 1"=w638, "Encoder pulses"=w641) -> ("Encoder velocity (pulse/s)"=w633:fxp<+/-,64,32>, "Shift Register out 2"=w635:i32, "Shift Register out 1"=w634:u32)  [unwired: 3 in]
    n353 = Multiply(x=w633, y=fxp<+/-,20,-5> 0.002499997615814209) -> (x*y=w631:fxp<+/-,64,27>)
    "Dy_d (M)" <- w631
    n354 = Multiply(x=w630, y=w631) -> (x*y=→"omega_y (M)":fxp<+/-,64,30>)
  }
  n355 = while "omega_y (T)" {
    shift-right: [w652] -> _
    shift-left: _ -> [w651]
    shift-right: [w646] -> _
    shift-left: _ -> [w650]
    shift-right: [w653] -> _
    shift-left: _ -> [w649]
    stop <- FALSE stop-if-true
    n356 = local read "Encoder Position_y"() -> (w652:i32)
    n357 = call "Tick Count7"() -> ("Tick Count(Ticks)"=w648:u32)
    n358 = call "omega_sub_Encoder_800ppr.vi"("mt0"="mt0_y", "omega_pre"=w650, "ticks_m_pre"=w649, "ticks"=w648, "count_pre"=w651, "count"=w652) -> ("ticks_m"=w653:u32, "mt"=→"mt_y":u32, "omega"=w646:fxp<+/-,20,9>)  [unwired: 3 in]
    "omega_y (T)" <- w646
    n359 = xnode ("High Throughput Multiply")("x"=fxp<+/-,26,1> 0.3183099031448364, "y"=w646) -> ("x*y"=→"Dy_d (T)":fxp<+/-,46,10>)
  }
  n360 = while "Velocity estiomation methods switch_y" {
    stop <- FALSE stop-if-true
    n361 = case shown="2" "Velocity Estimation_y" {
      tunnel: [w659 w660 w663] -> w656
      tunnel: [w658 w661 w662] -> w655
      frame 0, Default {
        n362 = local read "omega_y(M_avg)"() -> (w659:fxp<+/-,32,8>)
        n363 = local read "Dy_d (M_avg)"() -> (w658:fxp<+,32,8>)
      }
      frame 1 {
        n364 = local read "omega_y (M)"() -> (w660:fxp<+/-,32,8>)
        n365 = local read "Dy_d (M)"() -> (w661:fxp<+/-,32,8>)
      }
      frame 2 {
        n366 = local read "omega_y (T)"() -> (w663:fxp<+/-,20,9>)
        n367 = local read "Dy_d (T)"() -> (w662:fxp<+/-,32,8>)
      }
    }
    "omega_y (rad/s)" <- w656
    "Dy_d (mm/s)" <- w655
  }
  n368 = while "Integral and derivative_y" {
    shift-right: [w685] -> _
    shift-left: _ -> [w688]
    shift-right: [w674] -> _
    shift-left: _ -> [w665]
    shift-right: [w667] -> _
    shift-left: _ -> [w666]
    stop <- FALSE stop-if-true
    n369 = local read "Dy (mm)"() -> (w685:fxp<+/-,22,8>)
    n370 = local read "Dy_tolorence"() -> (w680:fxp<+/-,18,1>)
    n371 = local read "Dy_error"() -> (w677:fxp<+/-,37,10>)
    n372 = Subtract(x=w685, y=w688) -> (x-y=w687:fxp<+/-,23,9>)
    n373 = Absolute Value(x=w677) -> (abs(x)=w681:fxp<+,37,10>)
    n374 = Multiply(x=w687, y=fxp<+,7,10> 1000.0) -> (x*y=w684:fxp<+/-,30,19>)
    n375 = Greater?(x=w681, y=w680) -> (0:w679:bool)
    n376 = local read "Stop motor_y"() -> (w671:bool)
    n377 = Select(t=w677, s=w679, f=fxp<+,24,11> 0.0) -> (s? t:f=w674:fxp<+/-,39,12>)
    n378 = xnode "Butterworth Filter"("input data"=w684, "scaled coefficients"="scaled coefficients_Dy_dd") -> ("output data"=→"Dy_dd":fxp<+/-,34,23>)  [unwired: 1 in]
    n379 = Add(x=w665, y=w674) -> (x+y=w676:fxp<+/-,40,13>)
    n380 = Multiply(x=fxp<+/-,30,12> 0.000499725341796875, y=w676) -> (x*y=w673:fxp<+/-,64,24>)
    n381 = Select(t=fxp<+,1,1> 0.0, s=w671, f=fxp<+,1,1> 1.0) -> (s? t:f=w668:fxp<+,1,1>)
    n382 = Add(x=w673, y=w666) -> (x+y=w672:fxp<+/-,32,16>)
    n383 = Multiply(x=w672, y=w668) -> (x*y=w667:fxp<+/-,32,16>)
    "Dy_i" <- w667
    n384 = call "Wait4"("Count(uSec)"=u32 1000) -> ()  [unwired: 1 out]
  }
  n385 = while "Ramp gene._y" {
    stop <- FALSE stop-if-true
    n386 = flat-sequence {
      frame #0 {
        n387 = Divide(x="Dyr_end", y="Dyr_time") -> (x/y=→"Dyr_slope":fxp<+/-,64,30>)
      }
      frame #1 {
        n388 = local read "Time now_y (s)"() -> (w702:fxp<+,52,14>)
        n389 = while {
          tunnel: w702 -> [w707]
          stop <- FALSE stop-if-true
          n390 = local read "Time now_y (s)"() -> (w708:fxp<+,52,14>)
          n391 = local read "Dyr_slope"() -> (w705:fxp<+/-,32,10>)
          n392 = Subtract(x=w708, y=w707) -> (x-y=w706:fxp<+/-,53,15>)
          n393 = Multiply(x=w705, y=w706) -> (x*y=→"Dyr_ramp":fxp<+/-,64,24>)
        }
      }
    }
  }
